vi "ReadConfigFromFile.vi"(8 "error in (no error)":errorcluster, 11 "Camera_Prime95B in":refnum<class "Camera_Prime95B.lvclass">) -> (0 "error out":errorcluster, 3 "Camera_Prime95B out":refnum<class "Camera_Prime95B.lvclass">)   [LabVIEW 2020, in "Camera_Prime95B.lvlib" / "Camera_Prime95B.lvclass"]
uses:
  Camera_Prime95B.lvclass
  Camera_Prime95B.lvclass/Camera_Prime95B.ctl
  HAL Layer/Camera/Camera/Camera.lvclass
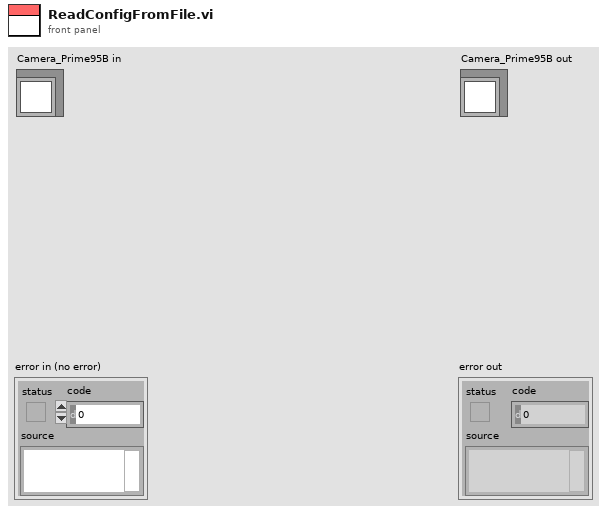
[diagram p1: front panel]
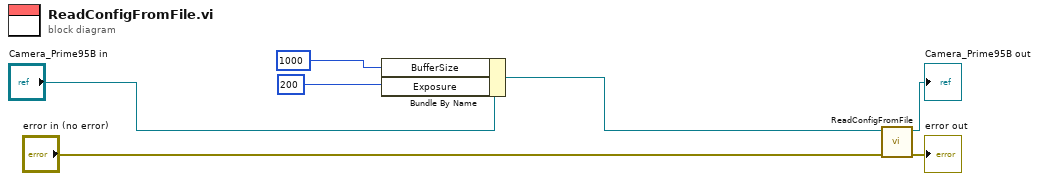
[diagram p0: block diagram]
diagram:
  n1 = Bundle By Name(cluster="Camera_Prime95B in", "BufferSize"=1000 ("Setting.BufferSize"), "Exposure"=200 ("Setting.Exposure")) -> (w1:refnum<class "Camera_Prime95B.lvclass">)
  n2 = call-parent "ReadConfigFromFile.vi"("error in (no error)"="error in (no error)", "Device in"=w1) -> ("error out"=→"error out":errorcluster, "Device out"=→"Camera_Prime95B out":refnum<class "Camera_Prime95B.lvclass">)  [unwired: 8 in]
